vi "init mc listbox stimulation status (subVI).vi"(0 "mc listbox refnum":refnum<vi>, 1 "colors cluster":T1={"background color (light grey)"=15132390, "font color (black)"=0, "selection color (yellow)"=16773465, "header background color (l blue)"=12833766}, 2 "font size (16)":u32=16, 3 "num visible rows (8)":u32=8, 5 "num solenoids (10)":i32=10, 11 "error in (no error)":errorcluster, 12 "cell width (35)":u32=35, 13 "description cell width (150)":u32=150) -> (4 "mc listbox refnum out":refnum<vi>, 15 "error out":errorcluster)   [LabVIEW 2021]
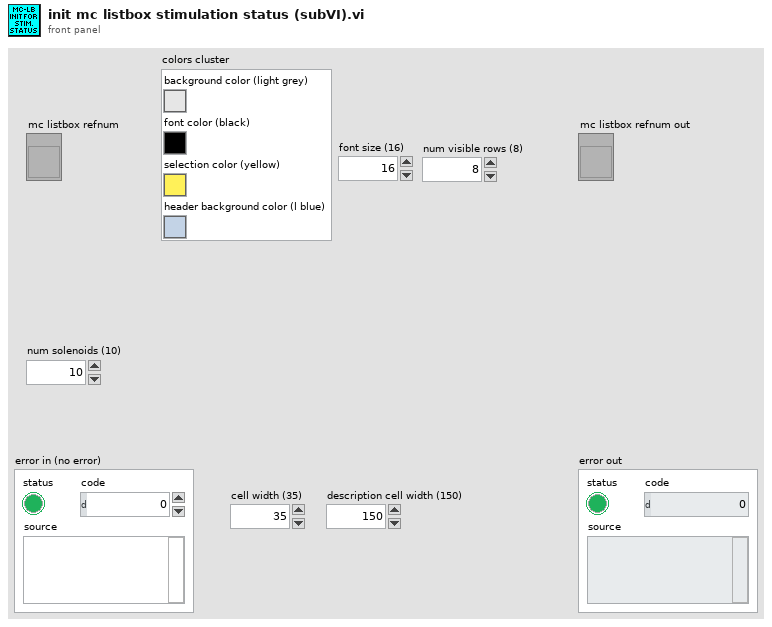
[diagram p1: front panel]
types:
  T1 = cluster{"background color (light grey)":u32, "font color (black)":u32, "selection color (yellow)":u32, "header background color (l blue)":u32}
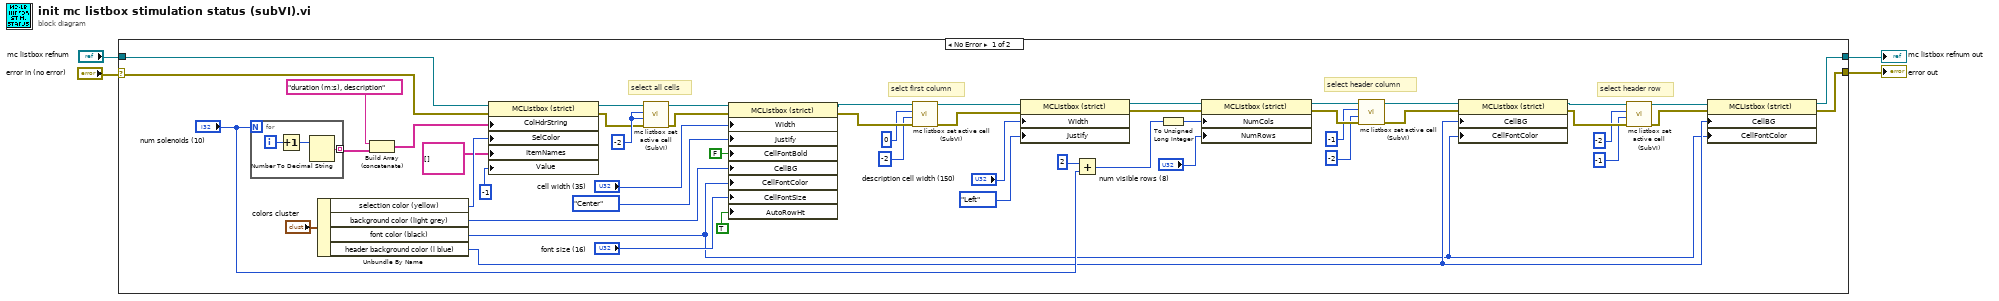
[diagram p0: block diagram]
diagram:
  n1 = case shown="No Error" "error in (no error)" {
    selector: "error in (no error)" -> [w18 w60]
    tunnel: [w38 w60] -> w4
    tunnel: [w37 w59] -> w3
    tunnel: "mc listbox refnum" -> [w23 w59]
    frame No Error {
      w55 = -2 ("row (0)")
      # "select all cells"
      # "select header column"
      # "select header row"
      # "selct first column"
      n2 = for {
        N: "num solenoids (10)" -> [_]
        tunnel: [w57] -> w21 mode=indexing
        i -> [w58]
        n3 = Increment(x=w58) -> (x+1=w56:i32)
        n4 = Number To Decimal String(number=w56) -> (decimal integer string=w57:string)  [unwired: 1 in]
      }
      n5 = Unbundle By Name("colors cluster") -> ("selection color (yellow)"=w8:u32, "background color (light grey)"=w9:u32, "font color (black)"=w10:u32, "header background color (l blue)"=w11:u32)
      n6 = Build Array (concatenate)("duration (m:s), description", w21) -> (w29:string[])
      n7 = property on="Property Node" class="MCListbox (strict)"(reference=w23, error in=w18, "ColHdrString"=w29, "SelColor"=w8, "ItemNames"=string[][] [] ("Item Names"), "Value"=-1) -> (reference out=w54:refnum<vi>, error out=w53:errorcluster)
      n8 = call "mc listbox set active cell (SubVI).vi"("error in (no error)"=w53, "row (0)"=w55, "column (0)"=w55, "multicolumn listbox refnum"=w54) -> ("error out"=w52:errorcluster, "multicolumn listbox refnum out"=w51:refnum<vi>)  [unwired: 6 in]
      n9 = property on="Property Node" class="MCListbox (strict)"(reference=w51, error in=w52, "Width"="cell width (35)", "Justify"=enum16{"Left", "Center", "Right"}."Center" ("Active Cell:Cell Justification"), "CellFontBold"=FALSE ("Active Cell:Cell Font:Bold"), "CellBG"=w9, "CellFontColor"=w10, "CellFontSize"="font size (16)", "AutoRowHt"=TRUE ("Autosizing Row Height")) -> (reference out=w47:refnum<vi>, error out=w48:errorcluster)
      n10 = call "mc listbox set active cell (SubVI).vi"("error in (no error)"=w48, "row (0)"=-2 ("Row"), "column (0)"=0 ("Column"), "multicolumn listbox refnum"=w47) -> ("error out"=w49:errorcluster, "multicolumn listbox refnum out"=w50:refnum<vi>)  [unwired: 6 in]
      n11 = property on="Property Node" class="MCListbox (strict)"(reference=w50, error in=w49, "Width"="description cell width (150)", "Justify"=enum16{"Left", "Center", "Right"}."Left" ("Active Cell:Cell Justification")) -> (reference out=w27:refnum<vi>, error out=w28:errorcluster)
      n12 = Add(x=2, y="num solenoids (10)") -> (x+y=w16:i32)
      n13 = To Unsigned Long Integer(number=w16) -> (unsigned 32bit integer=w14:u32)
      n14 = property on="Property Node" class="MCListbox (strict)"(reference=w27, error in=w28, "NumCols"=w14, "NumRows"="num visible rows (8)") -> (reference out=w34:refnum<vi>, error out=w33:errorcluster)
      n15 = call "mc listbox set active cell (SubVI).vi"("error in (no error)"=w33, "row (0)"=-2 ("Row"), "column (0)"=-1 ("Column"), "multicolumn listbox refnum"=w34) -> ("error out"=w35:errorcluster, "multicolumn listbox refnum out"=w36:refnum<vi>)  [unwired: 6 in]
      n16 = property on="Property Node" class="MCListbox (strict)"(reference=w36, error in=w35, "CellBG"=w11, "CellFontColor"=w10) -> (reference out=w41:refnum<vi>, error out=w42:errorcluster)
      n17 = call "mc listbox set active cell (SubVI).vi"("error in (no error)"=w42, "row (0)"=-1 ("Row"), "column (0)"=-2 ("Column"), "multicolumn listbox refnum"=w41) -> ("error out"=w43:errorcluster, "multicolumn listbox refnum out"=w44:refnum<vi>)  [unwired: 6 in]
      n18 = property on="Property Node" class="MCListbox (strict)"(reference=w44, error in=w43, "CellBG"=w11, "CellFontColor"=w10) -> (reference out=w37:refnum<vi>, error out=w38:errorcluster)
    }
    frame Error {
    }
  }
  "error out" <- w4
  "mc listbox refnum out" <- w3
